vi "Minimo.vi"(8 "error in (no error)":errorcluster, 10 "minimo":dbl, 11 "Counter ACQ in":refnum<class "Counter ACQ.lvclass">) -> (0 "error out":errorcluster, 3 "Counter ACQ out":refnum<class "Counter ACQ.lvclass">)   [LabVIEW 2019, in "Counter ACQ.lvlib" / "Counter ACQ.lvclass"]
uses:
  Counter ACQ.lvclass
  Counter ACQ.lvclass/Counter ACQ.ctl
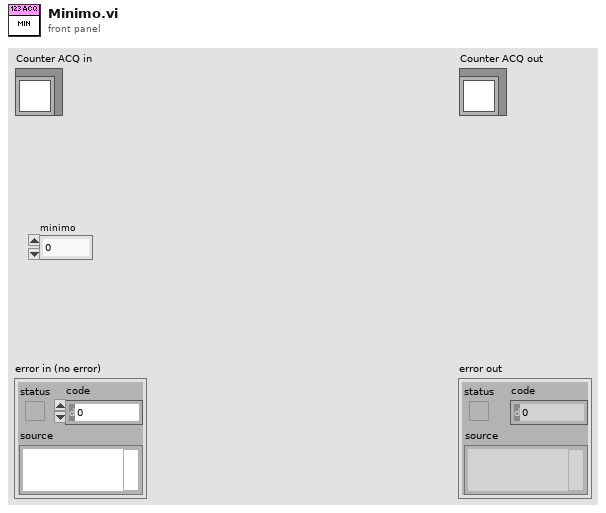
[diagram p1: front panel]
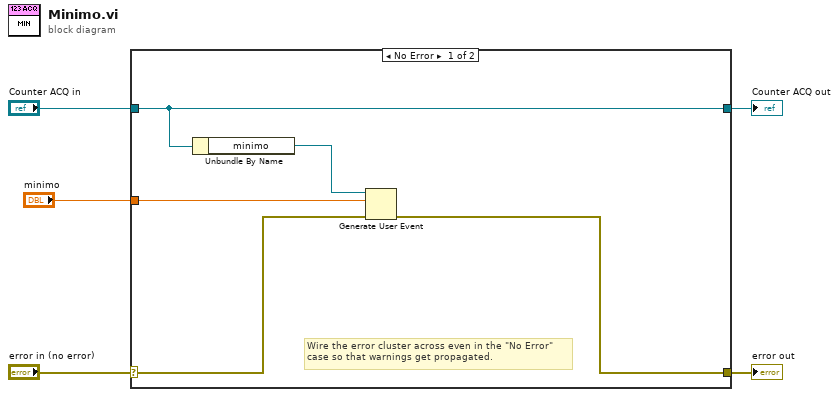
[diagram p0: block diagram]
diagram:
  n1 = case shown="No Error" "error in (no error)" {
    selector: "error in (no error)" -> [w7 w12]
    tunnel: [w6 w12] -> w4
    tunnel: [w10 w11] -> w2
    tunnel: "Counter ACQ in" -> [w10 w11]
    tunnel: "minimo" -> [w8 _]
    frame No Error {
      # "Wire the error cluster across even in the \"No Error\"\ncase so that warnings get propagated."
      n2 = Unbundle By Name(w10) -> ("minimo"=w9:refnum<user-event>)
      n3 = Generate User Event(user event=w9, event data cluster=w8, error in=w7) -> (error out=w6:errorcluster)  [unwired: 1 in, 1 out]
    }
    frame Error {
    }
  }
  "error out" <- w4
  "Counter ACQ out" <- w2
